vi "Read Canvas Ref.vi"(8 "error in (no error)":errorcluster, 11 "DrawingSystem in":refnum<class "DrawingSystem.lvclass">) -> (0 "error out":errorcluster, 2 "Canvas Ref":refnum<vi>, 3 "DrawingSystem out":refnum<class "DrawingSystem.lvclass">)   [LabVIEW 2022 SP3, in "DrawingSystem.lvclass"]
uses:
  DrawingSystem.lvclass
  DrawingSystem.lvclass/DrawingSystem.ctl
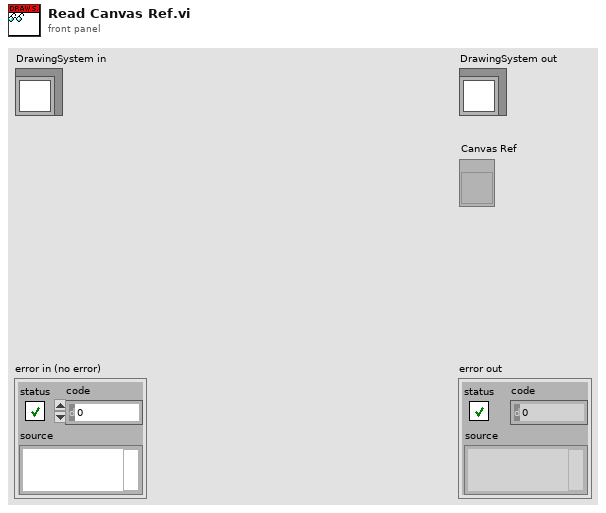
[diagram p1: front panel]
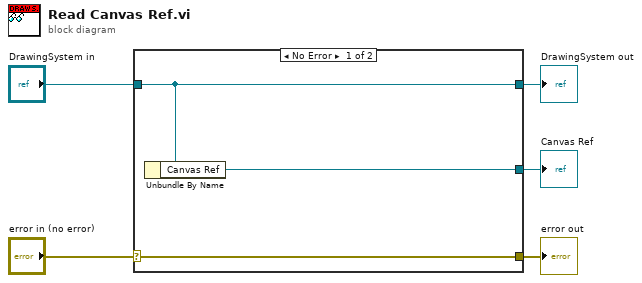
[diagram p0: block diagram]
diagram:
  n1 = case shown="No Error" "error in (no error)" {
    selector: "error in (no error)" -> [w8 w9]
    tunnel: [w8 w9] -> w4
    tunnel: [w7 w10] -> w2
    tunnel: "DrawingSystem in" -> [w7 w10]
    tunnel: [w6 _] -> w1
    frame No Error {
      n2 = Unbundle By Name(w7) -> ("Canvas Ref"=w6:refnum<vi>)
    }
    frame Error {
    }
  }
  "error out" <- w4
  "DrawingSystem out" <- w2
  "Canvas Ref" <- w1
